vi "documentary.vi"() -> ()   [LabVIEW 2014]
uses:
  <vilib>/addons/_office/excel.llb/Excel Get Data (dbl).vi
  <vilib>/Utility/NIReport.llb/NI_report.lvclass
  <vilib>/Utility/NIReport.llb/Excel/NI_Excel.lvclass
  <vilib>/addons/_office/NI_ReportGenerationToolkit.lvlib
panel:
  in  "Numeric":dbl
types:
  T1 = enum16{"Standard Report", "HTML", "Word", "Excel"}
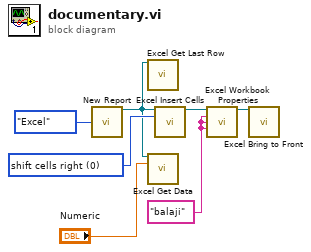
[diagram p0: block diagram]
diagram:
  w3 = "balaji" ("subject (\"\")")
  w6 = u16 0 items=["shift cells right", "shift cells down", "entire row", "entire column"] ("mode (entire row)")
  n1 = call <vilib>:"New Report.vi"("report type"=T1."Excel") -> ("report out"=w5:refnum<class "NI_report.lvclass">)  [unwired: 13 in, 1 out]
  n2 = call <vilib>:"Excel Get Last Row.vi"("report in"=w5) -> ()  [unwired: 12 in, 3 out]
  n3 = call-poly <vilib>:"Excel Get Data.vi"("report in"=w5, "data type"="Numeric") -> ()  [unwired: 11 in, 3 out]
  n4 = call <vilib>:"Excel Insert Cells.vi"("report in"=w5, "mode (entire row)"=w6) -> ("report out"=w4:refnum<class "NI_report.lvclass">)  [unwired: 12 in, 1 out]
  n5 = call <vilib>:"Excel Workbook Properties.vi"("report in"=w4, "subject (\"\")"=w3, "author (\"\")"=w3, "comments (\"\")"=w3) -> ("report out"=w2:refnum<class "NI_report.lvclass">)  [unwired: 8 in, 3 out]
  n6 = call <vilib>:"Excel Bring to Front.vi"("report in"=w2) -> ()  [unwired: 13 in, 2 out]
